vi "RichToFlatni_measurementlink_sessionmanagement_v1_ResolvedPinsOrRelays.vi"(5 "OutputClusterType":T1, 11 "InputCluster":T2) -> (3 "OutputCluster":T1)   [LabVIEW 2020, in "MeasurementLink Session Management Client.lvlib"]
uses:
  MeasurementLink Session Management Client.lvlib
  ni_measurementlink_sessionmanagement_v1_ResolvedPinsOrRelays.ctl
  ni_measurementlink_sessionmanagement_v1_ResolvedPinsOrRelays_Flat.ctl
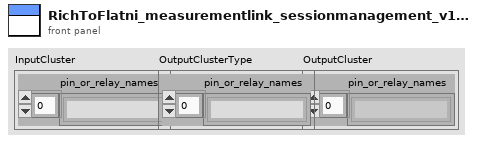
[diagram p1: front panel]
types:
  T1 = typedef "MeasurementLink Session Management Client.lvlib/ni_measurementlink_sessionmanagement_v1_ResolvedPinsOrRelays_Flat.ctl" = cluster{"pin_or_relay_names":string[]}
  T2 = typedef "MeasurementLink Session Management Client.lvlib/ni_measurementlink_sessionmanagement_v1_ResolvedPinsOrRelays.ctl" = cluster{"pin_or_relay_names":string[]}
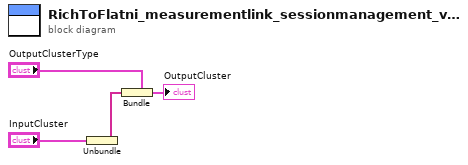
[diagram p0: block diagram]
diagram:
  n1 = Unbundle "Unbundle"("InputCluster") -> ("pin_or_relay_names"=w1:string[])
  n2 = Bundle "Bundle"(cluster="OutputClusterType", "pin_or_relay_names"=w1) -> (→"OutputCluster":T1)
